vi "set_all_logic_statements.vi"(8 "error in (no error)":errorcluster, 10 "All logic statements":string[](array[string]), 11 "VISA resource name":refnum<visa-resource-name>) -> (0 "error out":errorcluster, 3 "VISA resource name out":refnum<visa-resource-name>)   [LabVIEW 2018]
doc: "Update all logic statements."
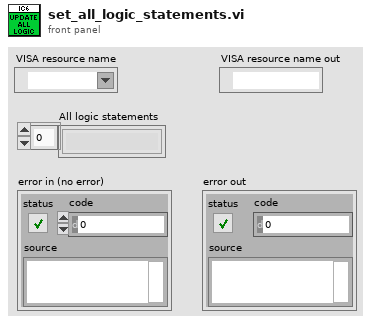
[diagram p1: front panel]
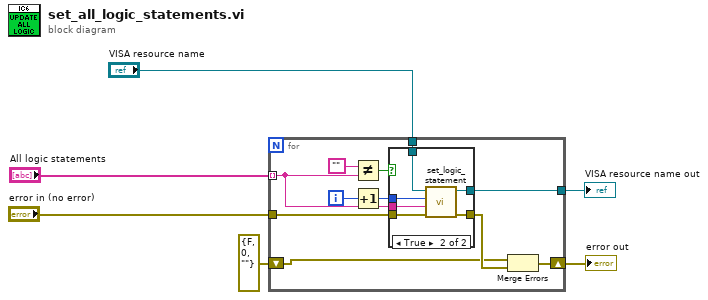
[diagram p0: block diagram]
diagram:
  n1 = for {
    tunnel: "All logic statements" -> [w10] mode=indexing
    tunnel: "VISA resource name" -> [w13]
    tunnel: [w11] -> w3
    tunnel: "error in (no error)" -> [w12]
    shift-right: [w9] -> w6
    shift-left: errorcluster {"status"=FALSE, "code"=0, "source"=""} ("error IO") -> [w7]
    i -> [w17]
    n2 = Not Equal?(x="", y=w10) -> (x != y?=w15:bool)
    n3 = Increment(x=w17) -> (x+1=w16:i32)
    n4 = case shown="True" w15 {
      tunnel: w16 -> [_ w24]
      tunnel: w10 -> [_ w23]
      tunnel: w13 -> [w19 w25]
      tunnel: [w19 w20] -> w11
      tunnel: w12 -> [w18 w22]
      tunnel: [w18 w21] -> w8
      frame False {
      }
      frame True {
        n5 = call "set_logic_statement.vi"("error in (no error)"=w22, "statement"=w23, "statement number"=w24, "VISA resource name"=w25) -> ("error out"=w21:errorcluster, "VISA resource name out"=w20:refnum<visa-resource-name>)  [unwired: 6 in]
      }
    }
    n6 = Merge Errors(w7, w8) -> (w9:errorcluster)
  }
  "error out" <- w6
  "VISA resource name out" <- w3
